vi "FieldByStepRotationForYakunin2.vi"() -> ()   [LabVIEW 2024]
panel:
  in  "New/Stop":bool
  in  "Rotator Position Max":dbl
  in  "Rotator position Min":dbl
  out "Direct Field Step:\nCurrent Value":dbl=0.1
  in  "Field Step Tab Control":enum32{"Direct Field", "Reciprocal Field"}(tab)
  in  "Direct Field Step (T)":dbl=0.1
  in  "DFS: Direct Field Step (T)":dbl=0.1
  in  "RFS: Reciprocal Field Step (1/T)":dbl=0.01
  in  "Threshold (T)":dbl=5.0
  in  "Calculate Setpoint":bool
  out "Power Supply State":string
  in  "Field:Rate [T/min]":dbl=0.2 min=0.0 max=0.6
  in  "Field:Final Setpoint":dbl min=-18.0 max=18.0
  out "Field: Current Value":dbl
  in  "stop":bool
  out "Field Runs":bool
  out "Field: Current Setpoint":dbl format="%.5f"
  out "Measurement Runs":bool
  in  "Steady Field":bool=TRUE
  # "Direct Field Step (DFS) will not be\nchanged below Threshold; while above: DFS=RFS*Field^2"
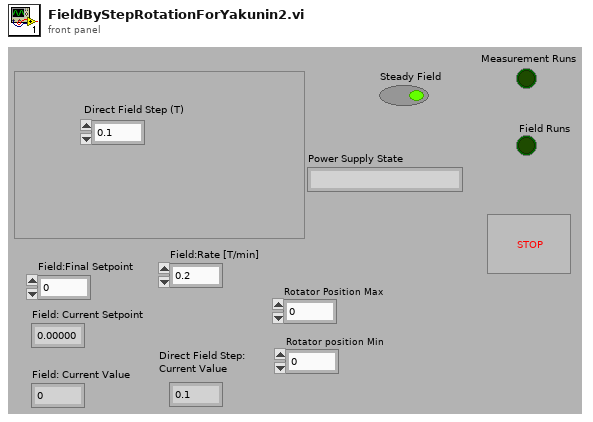
[diagram p1: front panel]
types:
  T1 = enum16{"No Response", "Ramping to programmed field ", "Holding at programmed field", "Paused", "Ramp Manual Up", "Ramp Manual Down", "Ramping to Zero", "QUENCH", "Heating Persistence Switch", "At Zero Current"}
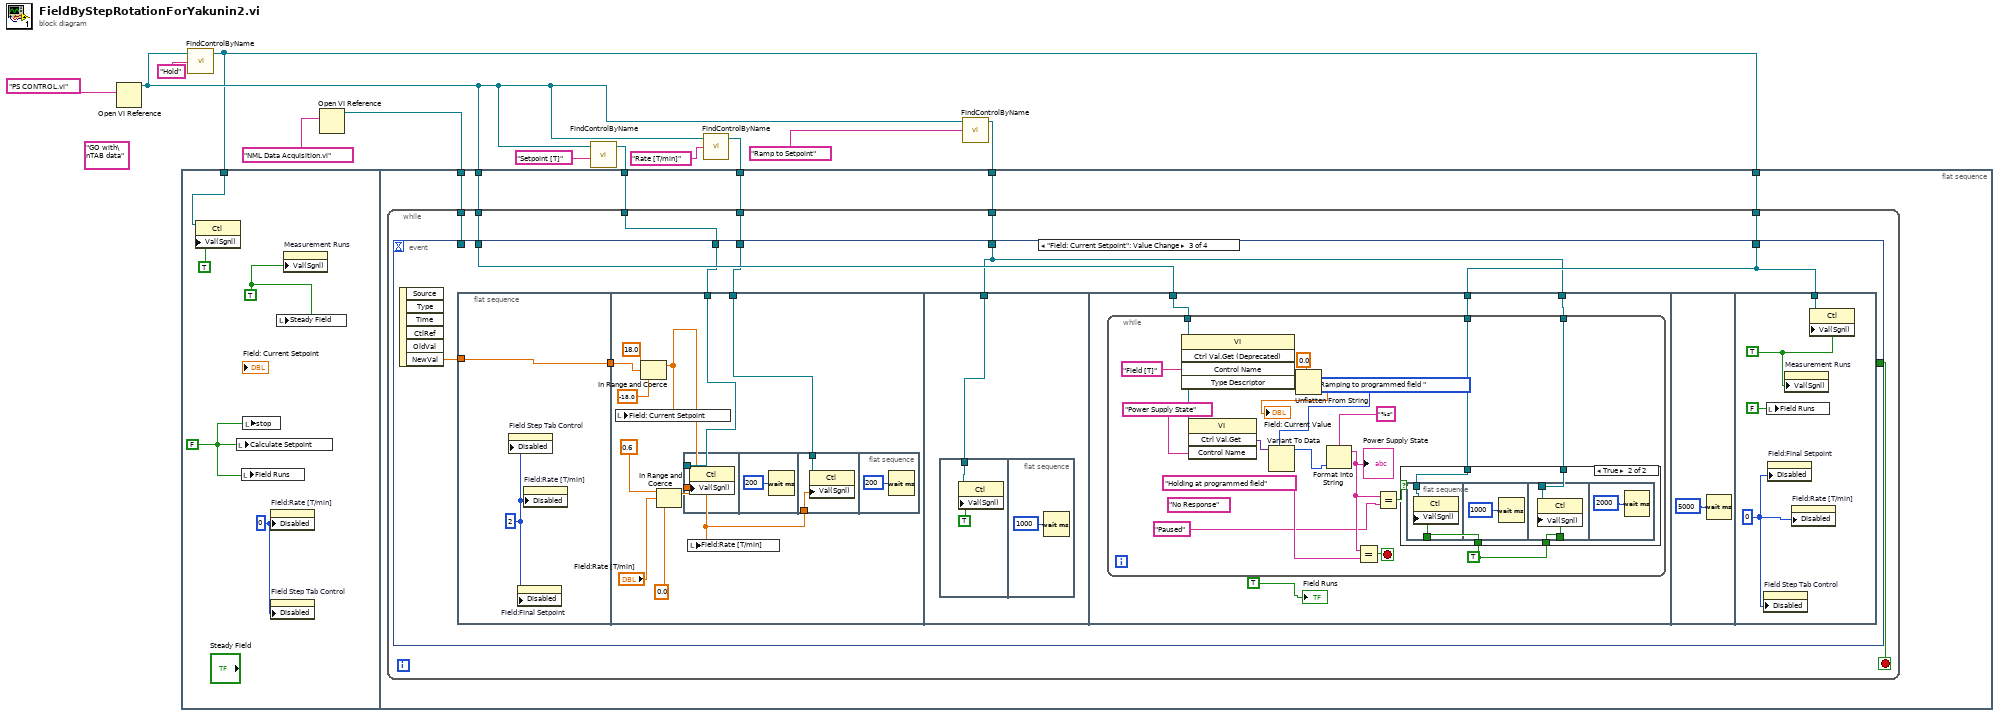
[diagram p0: block diagram]
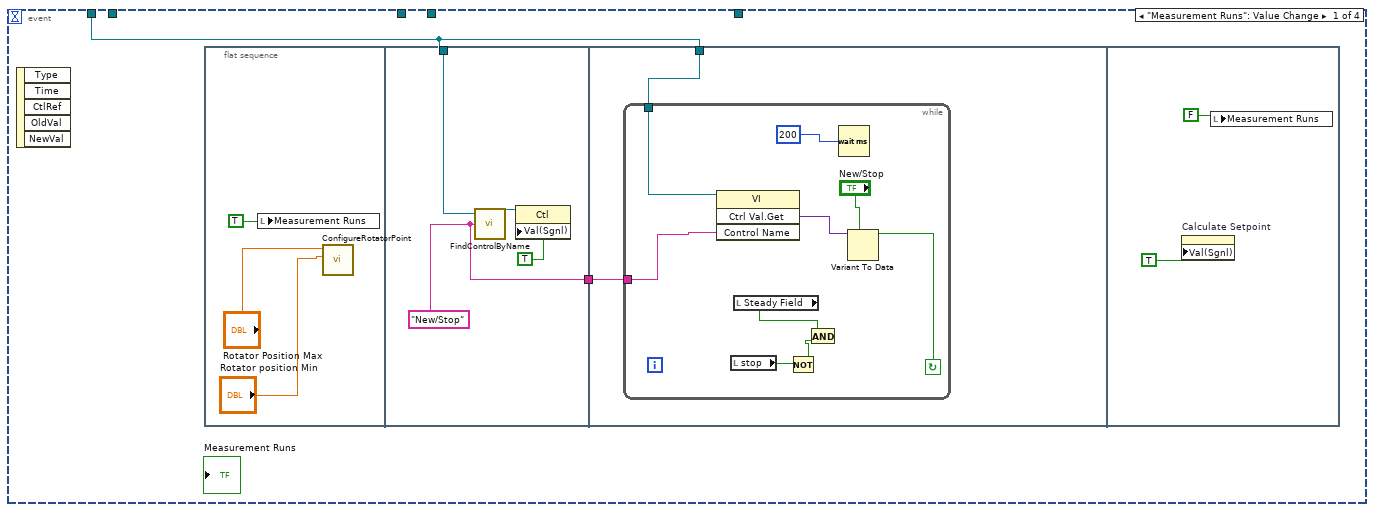
[diagram p2: hidden frame]
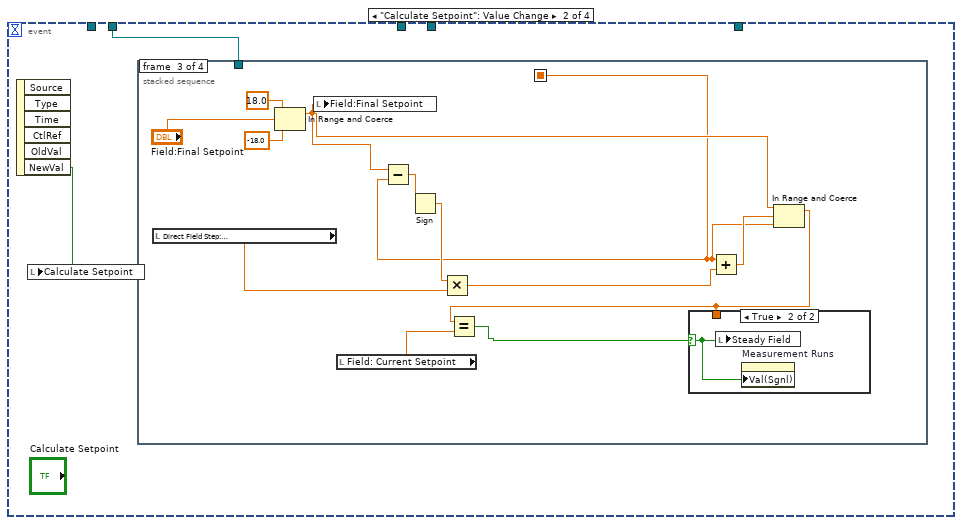
[diagram p3: hidden frame]
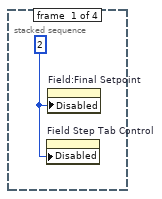
[diagram p4: hidden frame]
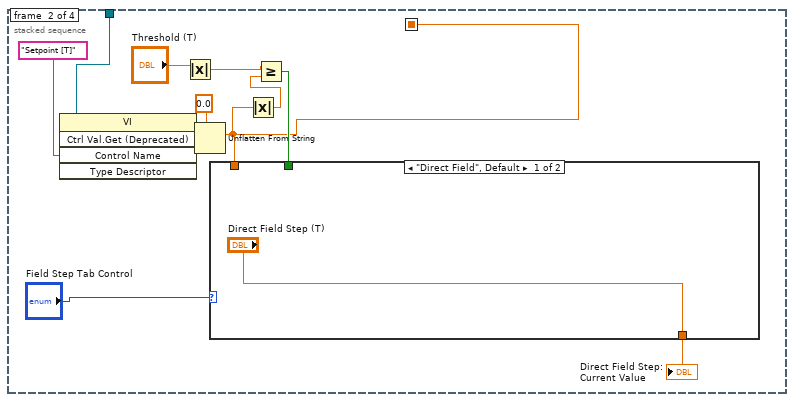
[diagram p5: hidden frame]
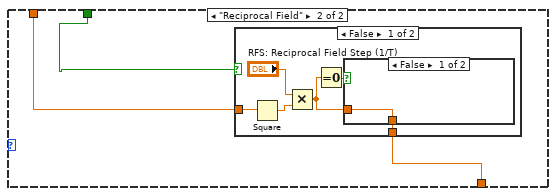
[diagram p6: hidden frame]
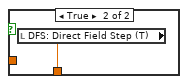
[diagram p7: hidden frame]
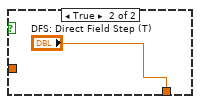
[diagram p8: hidden frame]
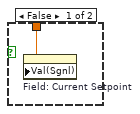
[diagram p9: hidden frame]
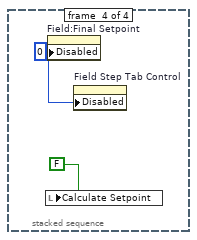
[diagram p10: hidden frame]
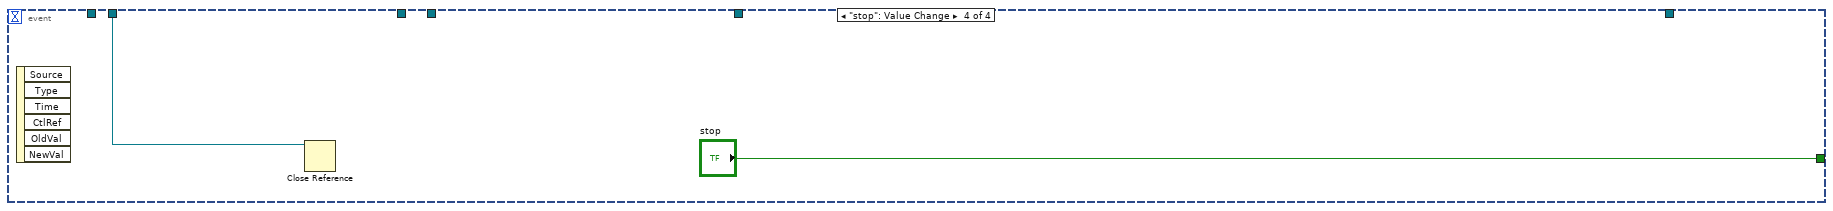
[diagram p12: hidden frame]
diagram:
  (unwired) "GO with\nTAB data" ("control name")
  n1 = Open VI Reference(vi path="PS CONTROL.vi") -> (vi reference=w4:refnum<vi>)  [unwired: 5 in, 1 out]
  n2 = flat-sequence {
    tunnel: w2 -> [w13]
    tunnel: w4 -> [w23]
    tunnel: w10 -> [w22]
    tunnel: w8 -> [w21]
    tunnel: w6 -> [w20]
    tunnel: w2 -> [w19]
    tunnel: w3 -> [w18]
    frame #0 {
      w15 = u8 0 ("Disabled")
      w17 = FALSE ("Boolean")
      w16 = TRUE ("Boolean")
      n3 = property class="Ctl"(reference=w13, "Val(Sgnl)"=TRUE ("Value (Signaling)")) -> ()  [unwired: 1 in, 2 out]
      n4 = local write "Calculate Setpoint"(w17) -> ()
      n5 = local write "Field Runs"(w17) -> ()
      n6 = local write "stop"(w17) -> ()
      n7 = property on="Field:Rate [T/min]" class="DigNum (strict)"("Disabled"=w15) -> ()  [unwired: 2 in, 2 out]
      n8 = property on="Field Step Tab Control" class="TabCtl (strict)"("Disabled"=w15) -> ()  [unwired: 2 in, 2 out]
      n9 = local write "Steady Field"(w16) -> ()
      n10 = property on="Measurement Runs" class="Bool (strict)"("Val(Sgnl)"=w16) -> ()  [unwired: 2 in, 2 out]
    }
    frame #1 {
      n11 = while {
        tunnel: w23 -> [w29]
        tunnel: w22 -> [w28]
        tunnel: w21 -> [w27]
        tunnel: w20 -> [w26]
        tunnel: w19 -> [w25]
        tunnel: w18 -> [w24]
        stop <- w30 stop-if-true
        n12 = event shown="[2] \"Field: Current Setpoint\": Value Change" {
          selector: _ -> [_ _ _ _]
          dyn-events: _ -> [_ _ _ _]
          timeout: _ -> [_ _ _ _]
          tunnel: [_ _ _ "stop"] -> w30
          tunnel: w29 -> [_ w53 w101 w163]
          tunnel: w28 -> [_ _ w100 _]
          tunnel: w27 -> [_ _ w99 _]
          tunnel: w26 -> [_ _ w97 _]
          tunnel: w25 -> [_ _ w98 _]
          tunnel: w24 -> [w31 _ _ _]
          event "Measurement Runs": Value Change {
            n13 = event-data() -> ()  [unwired: 1 in, 5 out]
            n14 = flat-sequence {
              tunnel: [w37] -> w32
              tunnel: w31 -> [w36]
              tunnel: w31 -> [w41]
              tunnel: w32 -> [w40]
              frame #0 {
                n15 = local write "Measurement Runs"(TRUE ("Measurement Test")) -> ()
                n16 = call "ConfigureRotatorPoint.vi"("Rotator Position Min"="Rotator position Min", "Rotator Position Max"="Rotator Position Max") -> ()  [unwired: 10 in]
              }
              frame #1 {
                w37 = "New/Stop" ("Control Name")
                n17 = call "FindControlByName.vi"("control name"=w37, "vi refnum"=w36) -> ("control refnum"=w39:refnum<vi>)  [unwired: 2 in, 1 out]
                n18 = property class="Ctl"(reference=w39, "Val(Sgnl)"=TRUE ("Value (Signaling)")) -> ()  [unwired: 1 in, 2 out]
              }
              frame #2 {
                n19 = while {
                  tunnel: w41 -> [w44]
                  tunnel: w40 -> [w43]
                  stop <- w45 continue-if-true
                  n20 = invoke class="VI" method="Ctrl Val.Get"(reference=w44, "Control Name"=w43) -> ("Get Control Value Variant"=w46:variant)  [unwired: 2 in, 3 out]
                  n21 = local read "stop"() -> (w49:bool)
                  n22 = local read "Steady Field"() -> (w47:bool)
                  n23 = Not(x=w49) -> (.not. x?=w48:bool)
                  n24 = And(x=w47, y=w48) -> ()  [unwired: 1 out]
                  n25 = Wait (ms)(milliseconds to wait=u32 200 ("millisecond timer value")) -> ()  [unwired: 1 out]
                  n26 = Variant To Data(type="New/Stop", Variant=w46) -> (data=w45:bool)  [unwired: 1 in, 1 out]
                }
              }
              frame #3 {
                n27 = property on="Calculate Setpoint" class="Bool (strict)"("Val(Sgnl)"=TRUE ("Value (Signaling)")) -> ()  [unwired: 2 in, 2 out]
                n28 = local write "Measurement Runs"(FALSE ("Measurement Test")) -> ()
              }
            }
          }
          event "Calculate Setpoint": Value Change {
            n29 = event-data() -> ("NewVal"=w54:bool)  [unwired: 1 in, 5 out]
            n30 = local write "Calculate Setpoint"(w54) -> ()
            n31 = stacked-sequence {
              seq-local: [_ w57 _ _] -> [_ _ w81 _]
              tunnel: w53 -> [_ w62 _ _]
              frame #0 {
                w55 = u8 2 ("Disabled")
                n32 = property on="Field Step Tab Control" class="TabCtl (strict)"("Disabled"=w55) -> ()  [unwired: 2 in, 2 out]
                n33 = property on="Field:Final Setpoint" class="DigNum (strict)"("Disabled"=w55) -> ()  [unwired: 2 in, 2 out]
              }
              frame #1 {
                n34 = invoke class="VI" method="Ctrl Val.Get (Deprecated)"(reference=w62, "Control Name"="Setpoint [T]") -> ("Get Control Value"=w64:string)  [unwired: 3 in, 4 out]
                n35 = Absolute Value(x="Threshold (T)") -> (abs(x)=w59:dbl)
                n36 = Unflatten From String(type=0.0, binary string=w64) -> (value=w57:dbl)  [unwired: 3 in, 2 out]
                n37 = Absolute Value(x=w57) -> (abs(x)=w60:dbl)
                n38 = Greater Or Equal?(x=w59, y=w60) -> (x >= y?=w58:bool)
                n39 = case shown="\"Direct Field\", Default" "Field Step Tab Control" {
                  tunnel: w58 -> [_ w70]
                  tunnel: w57 -> [_ w69]
                  tunnel: ["Direct Field Step (T)" w68] -> w56
                  frame "Direct Field", Default {
                  }
                  frame "Reciprocal Field" {
                    n40 = case shown="False" w70 {
                      tunnel: w69 -> [w74 _]
                      tunnel: [w71 "DFS: Direct Field Step (T)"] -> w68
                      frame False {
                        n41 = Square(x=w74) -> (x^2=w75:dbl)
                        n42 = Multiply(x="RFS: Reciprocal Field Step (1/T)", y=w75) -> (x*y=w72:dbl)
                        n43 = Equal To 0?(x=w72) -> (x = 0?=w73:bool)
                        n44 = case shown="False" w73 {
                          tunnel: w72 -> [w77 _]
                          tunnel: [w77 w78] -> w71
                          frame False {
                          }
                          frame True {
                            n45 = local read "DFS: Direct Field Step (T)"() -> (w78:dbl)
                          }
                        }
                      }
                      frame True {
                      }
                    }
                  }
                }
                "Direct Field Step:\nCurrent Value" <- w56
              }
              frame #2 {
                n46 = local read "Direct Field Step:\nCurrent Value"() -> (w80:dbl)
                n47 = In Range and Coerce(upper limit=18.0, x="Field:Final Setpoint", lower limit=-18.0) -> (coerced(x)=w82:dbl)  [unwired: 1 out]
                n48 = local write "Field:Final Setpoint"(w82) -> ()
                n49 = local read "Field: Current Setpoint"() -> (w86:dbl)
                n50 = Subtract(x=w82, y=w81) -> (x-y=w90:dbl)
                n51 = Sign(1:w90) -> (0:w89:dbl)
                n52 = Multiply(x=w89, y=w80) -> (x*y=w88:dbl)
                n53 = Add(x=w81, y=w88) -> (x+y=w87:dbl)
                n54 = In Range and Coerce(upper limit=w82, x=w87, lower limit=w81) -> (coerced(x)=w84:dbl)  [unwired: 1 out]
                n55 = Equal?(x=w84, y=w86) -> (x = y?=w85:bool)
                n56 = case shown="True" w85 {
                  selector: w85 -> [_ w94]
                  tunnel: w84 -> [w93 _]
                  frame False {
                    n57 = property on="Field: Current Setpoint" class="DigNum (strict)"("Val(Sgnl)"=w93) -> ()  [unwired: 2 in, 2 out]
                  }
                  frame True {
                    n58 = local write "Steady Field"(w94) -> ()
                    n59 = property on="Measurement Runs" class="Bool (strict)"("Val(Sgnl)"=w94) -> ()  [unwired: 2 in, 2 out]
                  }
                }
              }
              frame #3 {
                w95 = u8 0 ("Disabled")
                n60 = local write "Calculate Setpoint"(FALSE ("Calculate Setpoint")) -> ()
                n61 = property on="Field:Final Setpoint" class="DigNum (strict)"("Disabled"=w95) -> ()  [unwired: 2 in, 2 out]
                n62 = property on="Field Step Tab Control" class="TabCtl (strict)"("Disabled"=w95) -> ()  [unwired: 2 in, 2 out]
              }
            }
          }
          event "Field: Current Setpoint": Value Change {
            n63 = event-data() -> ("NewVal"=w103:dbl)  [unwired: 1 in, 5 out]
            n64 = flat-sequence {
              tunnel: w103 -> [w105]
              tunnel: [w105] -> w102
              tunnel: w102 -> [w115]
              tunnel: w100 -> [w107]
              tunnel: w99 -> [w109]
              tunnel: w97 -> [w122]
              tunnel: w101 -> [w129]
              tunnel: w98 -> [w127]
              tunnel: w97 -> [w126]
              tunnel: w98 -> [w159]
              frame #0 {
                w104 = u8 2 ("Disabled")
                n65 = property on="Field Step Tab Control" class="TabCtl (strict)"("Disabled"=w104) -> ()  [unwired: 2 in, 2 out]
                n66 = property on="Field:Final Setpoint" class="DigNum (strict)"("Disabled"=w104) -> ()  [unwired: 2 in, 2 out]
                n67 = property on="Field:Rate [T/min]" class="DigNum (strict)"("Disabled"=w104) -> ()  [unwired: 2 in, 2 out]
              }
              frame #1 {
                n68 = In Range and Coerce(upper limit=18.0, x=w115, lower limit=-18.0) -> (coerced(x)=w106:dbl)  [unwired: 1 out]
                n69 = local write "Field: Current Setpoint"(w106) -> ()
                n70 = In Range and Coerce(upper limit=0.6 ("x"), x="Field:Rate [T/min]", lower limit=0.0) -> (coerced(x)=w108:dbl)  [unwired: 1 out]
                n71 = flat-sequence {
                  tunnel: w107 -> [w117]
                  tunnel: w106 -> [w116]
                  tunnel: w109 -> [w120]
                  tunnel: w108 -> [w119]
                  frame #0 {
                    n72 = property class="Ctl"(reference=w117, "Val(Sgnl)"=w116) -> ()  [unwired: 1 in, 2 out]
                  }
                  frame #1 {
                    n73 = Wait (ms)(milliseconds to wait=u32 200 ("millisecond timer value")) -> ()  [unwired: 1 out]
                  }
                  frame #2 {
                    n74 = property class="Ctl"(reference=w120, "Val(Sgnl)"=w119) -> ()  [unwired: 1 in, 2 out]
                  }
                  frame #3 {
                    n75 = Wait (ms)(milliseconds to wait=u32 200 ("millisecond timer value")) -> ()  [unwired: 1 out]
                  }
                }
                n76 = local write "Field:Rate [T/min]"(w108) -> ()
              }
              frame #2 {
                n77 = flat-sequence {
                  tunnel: w122 -> [w123]
                  frame #0 {
                    n78 = property class="Ctl"(reference=w123, "Val(Sgnl)"=TRUE ("Value (Signaling)")) -> ()  [unwired: 1 in, 2 out]
                  }
                  frame #1 {
                    n79 = Wait (ms)(milliseconds to wait=u32 1000 ("millisecond timer value")) -> ()  [unwired: 1 out]
                  }
                }
              }
              frame #3 {
                n80 = while {
                  tunnel: w129 -> [w144]
                  tunnel: w127 -> [w133]
                  tunnel: w126 -> [w131]
                  stop <- w147 stop-if-true
                  w132 = TRUE
                  (unwired) "No Response"
                  n81 = invoke class="VI" method="Ctrl Val.Get (Deprecated)"(reference=w144, "Control Name"="Field [T]") -> ("Get Control Value"=w146:string)  [unwired: 3 in, 4 out]
                  n82 = invoke class="VI" method="Ctrl Val.Get"(reference=w144, "Control Name"="Power Supply State") -> ("Get Control Value Variant"=w140:variant)  [unwired: 2 in, 3 out]
                  n83 = Variant To Data(type=T1."Ramping to programmed field " ("Power Supply State 2"), Variant=w140) -> (data=w138:T1)  [unwired: 1 in, 1 out]
                  n84 = Unflatten From String(type=0.0, binary string=w146) -> (value=→"Field: Current Value":dbl)  [unwired: 3 in, 2 out]
                  n85 = Format Into String(format string="%s", w138) -> (resulting string=w136:string)  [unwired: 2 in, 1 out]
                  "Power Supply State" <- w136
                  n86 = Equal?(x=w136, y="Holding at programmed field") -> (x = y?=w147:bool)
                  n87 = Equal?(x=w136, y="Paused") -> (x = y?=w134:bool)
                  n88 = case shown="True" w134 {
                    tunnel: w133 -> [_ w151]
                    tunnel: w132 -> [_ w150]
                    tunnel: w132 -> [_ w149]
                    tunnel: w131 -> [_ w148]
                    frame False {
                    }
                    frame True {
                      n89 = flat-sequence {
                        tunnel: w151 -> [w153]
                        tunnel: w150 -> [w152]
                        tunnel: w148 -> [w156]
                        tunnel: w149 -> [w155]
                        frame #0 {
                          n90 = property class="Ctl"(reference=w153, "Val(Sgnl)"=w152) -> ()  [unwired: 1 in, 2 out]
                        }
                        frame #1 {
                          n91 = Wait (ms)(milliseconds to wait=u32 1000 ("millisecond timer value")) -> ()  [unwired: 1 out]
                        }
                        frame #2 {
                          n92 = property class="Ctl"(reference=w156, "Val(Sgnl)"=w155) -> ()  [unwired: 1 in, 2 out]
                        }
                        frame #3 {
                          n93 = Wait (ms)(milliseconds to wait=u32 2000 ("millisecond timer value")) -> ()  [unwired: 1 out]
                        }
                      }
                    }
                  }
                }
                "Field Runs" <- TRUE ("Field Test")
              }
              frame #4 {
                n94 = Wait (ms)(milliseconds to wait=u32 5000 ("millisecond timer value")) -> ()  [unwired: 1 out]
              }
              frame #5 {
                w160 = u8 0 ("Disabled")
                w161 = TRUE ("Value (Signaling)")
                n95 = property on="Field Step Tab Control" class="TabCtl (strict)"("Disabled"=w160) -> ()  [unwired: 2 in, 2 out]
                n96 = local write "Field Runs"(FALSE ("Field Test")) -> ()
                n97 = property on="Field:Final Setpoint" class="DigNum (strict)"("Disabled"=w160) -> ()  [unwired: 2 in, 2 out]
                n98 = property on="Measurement Runs" class="Bool (strict)"("Val(Sgnl)"=w161) -> ()  [unwired: 2 in, 2 out]
                n99 = property on="Field:Rate [T/min]" class="DigNum (strict)"("Disabled"=w160) -> ()  [unwired: 2 in, 2 out]
                n100 = property class="Ctl"(reference=w159, "Val(Sgnl)"=w161) -> ()  [unwired: 1 in, 2 out]
              }
            }
          }
          event "stop": Value Change {
            n101 = event-data() -> ()  [unwired: 1 in, 6 out]
            n102 = Close Reference(reference=w163) -> ()  [unwired: 1 in, 1 out]
          }
        }
      }
    }
  }
  n103 = call "FindControlByName.vi"("control name"="Hold" ("Control Name"), "vi refnum"=w4) -> ("control refnum"=w2:refnum<vi>)  [unwired: 2 in, 1 out]
  n104 = Open VI Reference(vi path="NML Data Acquisition.vi") -> (vi reference=w3:refnum<vi>)  [unwired: 5 in, 1 out]
  n105 = call "FindControlByName.vi"("control name"="Setpoint [T]" ("Control Name"), "vi refnum"=w4) -> ("control refnum"=w10:refnum<vi>)  [unwired: 2 in, 1 out]
  n106 = call "FindControlByName.vi"("control name"="Rate [T/min]" ("Control Name"), "vi refnum"=w4) -> ("control refnum"=w8:refnum<vi>)  [unwired: 2 in, 1 out]
  n107 = call "FindControlByName.vi"("control name"="Ramp to Setpoint" ("Control Name"), "vi refnum"=w4) -> ("control refnum"=w6:refnum<vi>)  [unwired: 2 in, 1 out]
